vi "solar_voy TCP Read.vi"(7 "Setup":T1, 8 "error in (no error)":errorcluster, 9 "timeout ms (-1)":i32=-1, 10 "Connection ID":refnum<k5>, 11 "Voyager Refnum in":T2) -> (0 "error out":errorcluster, 1 "ID":u16, 2 "TCP Data":string, 3 "Voyager Refnum out":T2)   [LabVIEW 2018]
doc: "This wait for the next TCP message to read specified by the Voyager interface header."
uses:
  solar_voy_ctl Port Setup.ctl
  solar_voy_ctl Voyager Refnum.ctl
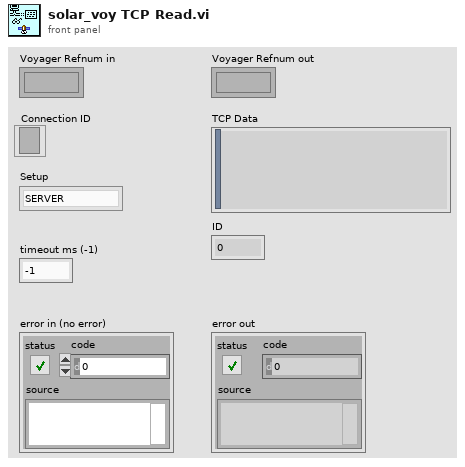
[diagram p1: front panel]
types:
  T1 = typedef "solar_voy_ctl Port Setup.ctl" = enum8{"SERVER", "CLIENT", "SERVER_CMD", "SERVER_TLM"}
  T2 = typedef "solar_voy_ctl Voyager Refnum.ctl" = refnum<k1>
  T3 = typedef "solar_voy_ctl Voyager.ctl" = cluster{"PACKETS":T4[], "COSMOS_Root":path, "CMD_HDR":T9, "TLM_HDR":T9, "TCPs":T10[], "VoyagerIDOffset":cluster{"VoyagerIDOffset":u16[], "Target Names":string[]}}
  T4 = typedef "solar_voy_def_ctl PACKET.ctl" = cluster{"PACKET_ID":T5, "ENDIAN":enum8{"BIG", "LITTLE"}, "DESC":string, "HZRD":bool, "ITEMS":T6[], "NoExport":bool, "last_time":timestamp, "last_count":u32, "last_data":string}
  T5 = typedef "solar_voy_def_ctl PACKET_ID.ctl" = cluster{"ID":u16, "CMD":enum8{"CMD", "TLM"}, "TARGET":string, "PACKET":string}
  T6 = typedef "solar_voy_def_ctl ITEM.ctl" = cluster{"NAME":string, "OFFSET":i32, "SIZE":i32, "TYPE":T7, "EACH_SIZE":i32, "LVTYPE":T8, "MIN":dbl, "MAX":dbl, "DEFAULT":string, "DESC":string, "ID":bool, "MODIFIERS":variant, "last_value":variant}
  T7 = typedef "solar_voy_def_ctl ITEM TYPE.ctl" = enum8{"BLOCK", "INT", "UINT", "FLOAT", "STRING"}
  T8 = typedef "solar_type Item Type.ctl" = enum16{"NULL", "UNKNOWN", "CLUSTER", "I8", "I16", "I32", "I64", "U8", "U16", "U32", "U64", "U8_ENUM", "U16_ENUM", "U32_ENUM", "SGL", "DBL", "BOOLEAN", "STRING", "PATH", "VISA", "TAG", "TIME", "I8_1D", "I16_1D", "I32_1D", "I64_1D", "U8_1D", "U16_1D", "U32_1D", "U64_1D", "U8_ENUM_1D", "U16_ENUM_1D", "U32_ENUM_1D", "SGL_1D", "DBL_1D", "BOOLEAN_1D", "STRING_1D", "PATH_1D", "VISA_1D", "TAG_1D", "TIME_1D", "I8_2D", "I16_2D", "I32_2D", "I64_2D", "U8_2D", "U16_2D", "U32_2D", "U64_2D", "U8_ENUM_2D", "U16_ENUM_2D", "U32_ENUM_2D", "SGL_2D", "DBL_2D", "BOOLEAN_2D", "STRING_2D", "PATH_2D", "VISA_2D", "TAG_2D", "TIME_2D"}
  T9 = typedef "solar_voy_def_ctl HDR.ctl" = cluster{"ITEMS":T6[], "LENGTH_NAME":string, "LENGTH_VALUE_OFFSET":i32, "ID_NAME":string, "ENDIAN":enum8{"BIG", "LITTLE"}, "GUID_NAME":string, "DEFAULT_TARGET":string, "DEFAULT_PACKET":string, "DEFAULT_ERROR":string}
  T10 = typedef "solar_voy_ctl TCP.ctl" = cluster{"Connected":bool, "Port":u16, "Listener":refnum<k5>, "ServerIP":string, "TCP":refnum<k5>, "Setup":T1, "VIRefnum":refnum<vi>, "TARGETS_CMD":string[], "TARGETS_TLM":string[]}
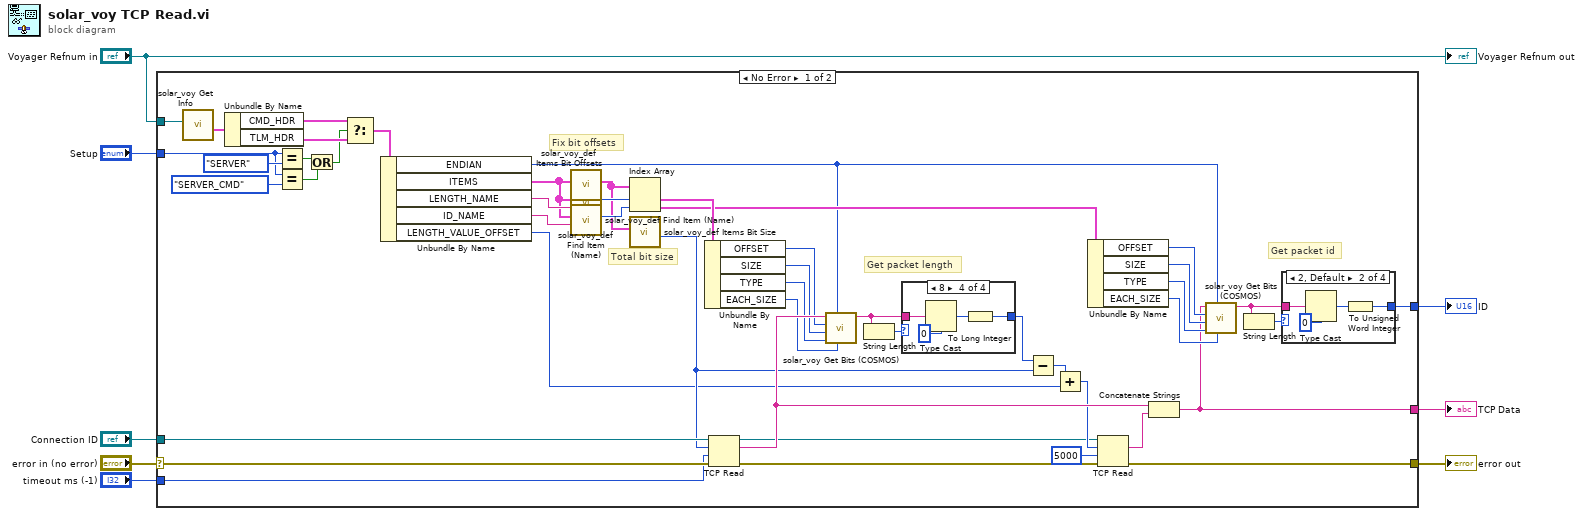
[diagram p0: block diagram]
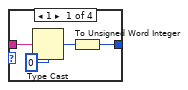
[diagram p2: hidden frame]
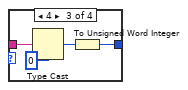
[diagram p3: hidden frame]
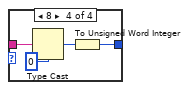
[diagram p4: hidden frame]
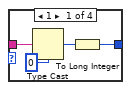
[diagram p5: hidden frame]
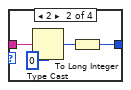
[diagram p6: hidden frame]
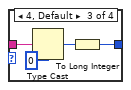
[diagram p7: hidden frame]
diagram:
  n1 = case shown="No Error" "error in (no error)" {
    selector: "error in (no error)" -> [w46 w89]
    tunnel: [w56 w89] -> w8
    tunnel: "Connection ID" -> [w47 _]
    tunnel: "timeout ms (-1)" -> [w45 _]
    tunnel: "Voyager Refnum in" -> [w44 _]
    tunnel: "Setup" -> [w11 _]
    tunnel: [w20 _] -> w2
    tunnel: [w19 _] -> w1
    frame No Error {
      # "Total bit size"
      # "Get packet id"
      # "Get packet length"
      # "Fix bit offsets"
      n2 = call "solar_voy Get Info.vi"("Voyager Refnum"=w44) -> ("Voyager"=w43:T3)  [unwired: 8 in, 2 out]
      n3 = Unbundle By Name(w43) -> ("CMD_HDR"=w18:T9, "TLM_HDR"=w17:T9)
      n4 = Equal?(x=w11, y=solar_voy_ctl_Port_Setup."SERVER") -> (x = y?=w14:bool)
      n5 = Equal?(x=w11, y=solar_voy_ctl_Port_Setup."SERVER_CMD") -> (x = y?=w9:bool)
      n6 = Or(x=w14, y=w9) -> (x .or. y?=w12:bool)
      n7 = Select(t=w18, s=w12, f=w17) -> (s? t:f=w16:T9)
      n8 = Unbundle By Name(w16) -> ("ENDIAN"=w15:enum8{"BIG", "LITTLE"}, "ITEMS"=w24:T6[], "LENGTH_NAME"=w42:string, "ID_NAME"=w41:string, "LENGTH_VALUE_OFFSET"=w31:i32)
      n9 = call "solar_voy_def Items Bit Offsets.vi"("ITEMS in"=w24) -> ("ITEMS with Bit Offsets"=w22:T6[])  [unwired: 9 in, 1 out]
      n10 = call "solar_voy_def Find Item (Name).vi"("ITEM_NAME"=w42, "ITEMS"=w24) -> ("Index"=w40:i32)  [unwired: 9 in]
      n11 = call "solar_voy_def Find Item (Name).vi"("ITEM_NAME"=w41, "ITEMS"=w24) -> ("Index"=w39:i32)  [unwired: 9 in]
      n12 = Index Array(array=w22, index #1=w40, index #2=w39) -> (element #1=w38:T6, element #2=w25:T6)
      n13 = call "solar_voy_def Items Bit Size.vi"("ITEMS"=w22) -> ("Byte Size"=w37:i32)  [unwired: 9 in, 1 out]
      n14 = Unbundle By Name(w38) -> ("OFFSET"=w36:i32, "SIZE"=w34:i32, "TYPE"=w35:T7, "EACH_SIZE"=w23:i32)
      n15 = TCP Read(connection ID=w47, bytes to read=w37, error in (no error)=w46, 9:w45) -> (connection ID out=w51:refnum<k5>, data out=w55:string, error out=w50:errorcluster)  [unwired: 1 out]
      n16 = call "solar_voy Get Bits (COSMOS).vi"("Bit Element Size (Array only)"=w23, "Endian (BIG)"=w15, "COSMOS TYPE"=w35, "Bit Size"=w34, "Bit Offset"=w36, "COSMOS Data"=w55) -> ("LabVIEW Flattened Value"=w32:string)  [unwired: 4 in, 1 out]
      n17 = String Length(string=w32) -> (length=w33:i32)
      n18 = case shown="8" w33 {
        tunnel: w32 -> [w76 w80 w84 w88]
        tunnel: [w73 w77 w81 w85] -> w49
        frame 1 {
          n19 = Type Cast(type=u8 0, x=w76) -> (*(type *) &x=w74:u8)
          n20 = To Long Integer(number=w74) -> (32bit integer=w73:i32)
        }
        frame 2 {
          n21 = Type Cast(type=u16 0, x=w80) -> (*(type *) &x=w78:u16)
          n22 = To Long Integer(number=w78) -> (32bit integer=w77:i32)
        }
        frame 4, Default {
          n23 = Type Cast(type=u32 0, x=w84) -> (*(type *) &x=w82:u32)
          n24 = To Long Integer(number=w82) -> (32bit integer=w81:i32)
        }
        frame 8 {
          n25 = Type Cast(type=u64 0, x=w88) -> (*(type *) &x=w86:u64)
          n26 = To Long Integer(number=w86) -> (32bit integer=w85:i32)
        }
      }
      n27 = Subtract(x=w49, y=w37) -> (x-y=w48:i32)
      n28 = Add(x=w48, y=w31) -> (x+y=w52:i32)
      n29 = Unbundle By Name(w25) -> ("OFFSET"=w26:i32, "SIZE"=w28:i32, "TYPE"=w27:T7, "EACH_SIZE"=w21:i32)
      n30 = TCP Read(connection ID=w51, bytes to read=w52, error in (no error)=w50, 9:5000 ("timeout ms (25000)")) -> (data out=w54:string, error out=w56:errorcluster)  [unwired: 2 out]
      n31 = Concatenate Strings(w55, w54) -> (w20:string)
      n32 = call "solar_voy Get Bits (COSMOS).vi"("Bit Element Size (Array only)"=w21, "Endian (BIG)"=w15, "COSMOS TYPE"=w27, "Bit Size"=w28, "Bit Offset"=w26, "COSMOS Data"=w20) -> ("LabVIEW Flattened Value"=w30:string)  [unwired: 4 in, 1 out]
      n33 = String Length(string=w30) -> (length=w29:i32)
      n34 = case shown="2, Default" w29 {
        tunnel: w30 -> [w60 w64 w68 w72]
        tunnel: [w57 w61 w65 w69] -> w19
        frame 1 {
          n35 = Type Cast(type=u8 0, x=w60) -> (*(type *) &x=w58:u8)
          n36 = To Unsigned Word Integer(number=w58) -> (unsigned 16bit integer=w57:u16)
        }
        frame 2, Default {
          n37 = Type Cast(type=u16 0, x=w64) -> (*(type *) &x=w62:u16)
          n38 = To Unsigned Word Integer(number=w62) -> (unsigned 16bit integer=w61:u16)
        }
        frame 4 {
          n39 = Type Cast(type=u32 0, x=w68) -> (*(type *) &x=w66:u32)
          n40 = To Unsigned Word Integer(number=w66) -> (unsigned 16bit integer=w65:u16)
        }
        frame 8 {
          n41 = Type Cast(type=u64 0, x=w72) -> (*(type *) &x=w70:u64)
          n42 = To Unsigned Word Integer(number=w70) -> (unsigned 16bit integer=w69:u16)
        }
      }
    }
    frame Error {
    }
  }
  "TCP Data" <- w2
  "error out" <- w8
  "ID" <- w1
  "Voyager Refnum out" <- "Voyager Refnum in"
